vi "setDigitalOutput.vi"(0 "Controller in":refnum<class "_Controller.lvclass">, 2 "digital_output_ch":T1, 3 "dig_out_value":bool, 5 "error in (no error)":errorcluster) -> (14 "Controller out":refnum<class "_Controller.lvclass">, 17 "response":string, 18 "success?":bool, 19 "error out":errorcluster)   [LabVIEW 2013, in "classes.lvlib" / "_Controller.lvclass"]
doc: "Sets the DO state of a given Digital Output channel\n\nProduced By:\n\n<B>Kod Integrations, LLC</B>\n4835 Marianne Drive\nMount Airy, MD 21771\nhttp://www.kodintegrations.com\nemail: info@kodintegrations.com\nphone: (240) 687-1288"
uses:
  _Controller.lvclass
  digital_output.ctl
  commands.ctl
  common.lvlib
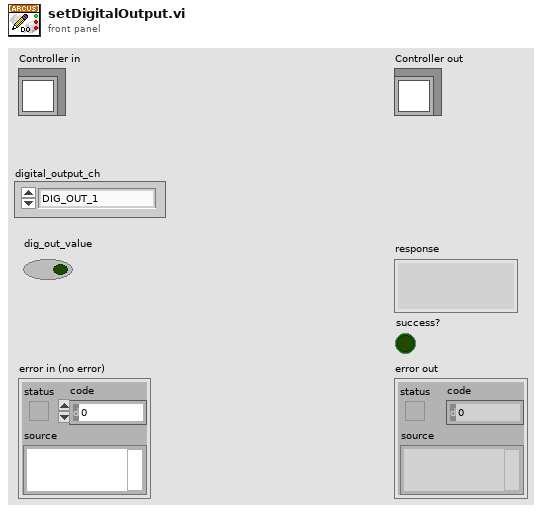
[diagram p1: front panel]
types:
  T1 = typedef "common.lvlib/digital_output.ctl" = enum16{"DIG_OUT_1", "DIG_OUT_2", "DIG_OUT_3", "DIG_OUT_4", "DIG_OUT_5", "DIG_OUT_6", "DIG_OUT_7", "DIG_OUT_8"}
  T2 = typedef "common.lvlib/commands.ctl" = enum16{"clear error", "constant jog(-)", "constant jog(+)", "get acceleration", "get actual current", "get device name", "get digital input status", "get digital inputs status", "get digital output status", "get digital outputs status", "get firmware ver", "get high speed", "get idle current", "get low speed", "get micro step", "get motor status", "get move mode", "get polarity", "get position", "get product id", "get power status", "get run current", "get status", "home(-)", "home(+)", "move to position", "power down", "power up", "set acceleration", "set device id", "set digital output", "set digital outputs", "set high speed", "set idle current", "set low speed", "set move mode absolute", "set move mode increment", "set polarity", "set position", "set run current", "stop immediate", "stop slow", "store to memory"}
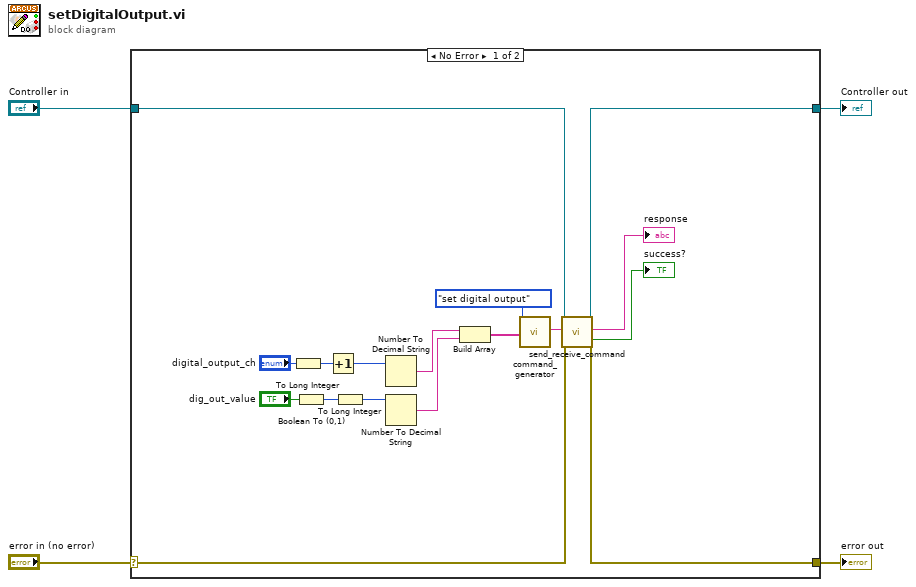
[diagram p0: block diagram]
diagram:
  n1 = case shown="No Error" "error in (no error)" {
    selector: "error in (no error)" -> [w7 w23]
    tunnel: [w6 w23] -> w3
    tunnel: [w10 w22] -> w1
    tunnel: "Controller in" -> [w11 w22]
    frame No Error {
      n2 = To Long Integer(number="digital_output_ch") -> (32bit integer=w16:i32)
      n3 = Boolean To (0,1)(Boolean="dig_out_value") -> (0, 1=w18:i16)
      n4 = Increment(x=w16) -> (x+1=w14:i32)
      n5 = To Long Integer(number=w18) -> (32bit integer=w17:i32)
      n6 = Number To Decimal String(number=w14) -> (decimal integer string=w21:string)  [unwired: 1 in]
      n7 = Number To Decimal String(number=w17) -> (decimal integer string=w20:string)  [unwired: 1 in]
      n8 = Build Array(w21, w20) -> (w12:string[])
      n9 = call "command_generator.vi"("cmd (in)"=commands."set digital output" ("command"), "params (in)"=w12) -> ("ASCII_cmd (out)"=w9:string)  [unwired: 17 in]
      n10 = call "send_receive_command.vi"("reference (in)"=w11, "ASCII Command (in)"=w9, "error in (no error)"=w7) -> ("reference (out)"=w10:refnum<class "_Controller.lvclass">, "response (out)"=→"response":string, "success?"=→"success?":bool, "error out"=w6:errorcluster)  [unwired: 12 in, 1 out]
    }
    frame Error {
    }
  }
  "error out" <- w3
  "Controller out" <- w1
